vi "_PC_Pub_AddTabSpaceInString.vi"(8 "error in (no error)":errorcluster, 10 "Position in":i32, 11 "String in":string) -> (0 "error out":errorcluster, 2 "Position out":i32, 3 "String out":string)   [LabVIEW 2018]
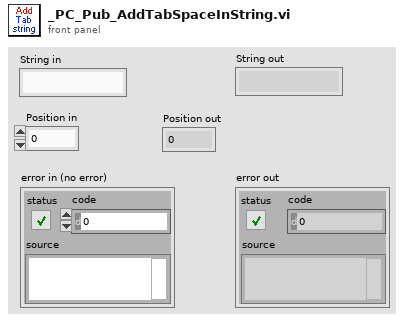
[diagram p1: front panel]
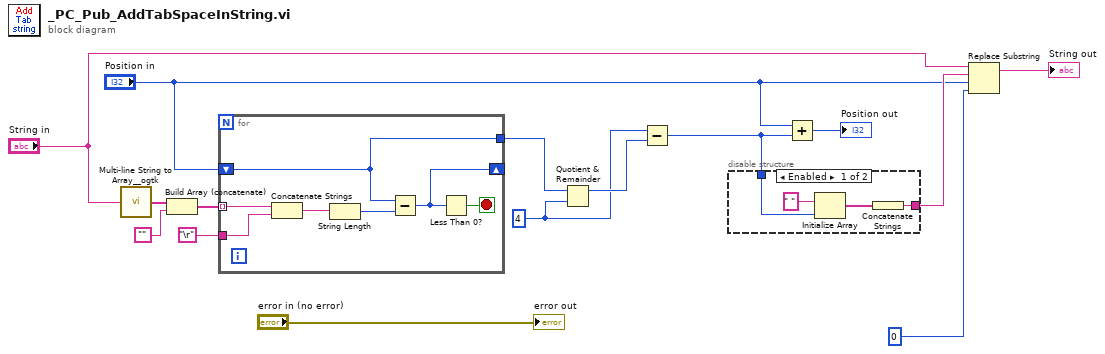
[diagram p0: block diagram]
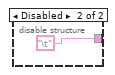
[diagram p2: hidden frame]
diagram:
  w9 = 4 ("y")
  n1 = call <userlib>:"Multi-line String to Array__ogtk.vi"("string"="String in") -> ("lines"=w6:string[])
  n2 = Build Array (concatenate)(w6, "") -> (w3:string[])
  n3 = for {
    shift-right: [w22] -> _
    shift-left: "Position in" -> [w21]
    tunnel: [w21] -> w11
    tunnel: w3 -> [w19] mode=indexing
    tunnel: "\r" -> [w16]
    stop <- w20 stop-if-true
    n4 = Concatenate Strings(w19, w16) -> (w17:string)
    n5 = String Length(string=w17) -> (length=w18:i32)
    n6 = Subtract(x=w21, y=w18) -> (x-y=w22:i32)
    n7 = Less Than 0?(x=w22) -> (x < 0?=w20:bool)
  }
  n8 = Quotient & Remainder(x=w11, y=w9) -> (x-y*floor(x/y)=w10:i32)  [unwired: 1 out]
  n9 = Subtract(x=w9, y=w10) -> (x-y=w7:i32)
  n10 = disable-structure shown="Enabled" {
    disable-tunnel: [w24 "\t"] -> w12
    disable-tunnel: w7 -> [w23 _]
    frame Enabled {
      n11 = Initialize Array(" ", w23) -> (w26:string[])
      n12 = Concatenate Strings(w26) -> (w24:string)
    }
    frame Disabled {
    }
  }
  n13 = Add(x="Position in", y=w7) -> (x+y=→"Position out":i32)
  n14 = Replace Substring(2:0 ("length (len. of substring)"), 3:"Position in", 4:w12, 5:"String in") -> (1:→"String out":string)  [unwired: 1 out]
  "error out" <- "error in (no error)"
